vi "new Sub Address.vi"(6 "direction (Tx)":i32(ring) items=["Tx", "Rx"], 7 "messageBufferIDRef (-1)":i32=-1, 8 "error in":errorcluster, 9 "subAddress":i8, 10 "SubAddress Config":T1 {"elapseMinOrMax" items=["A", "B", "AB", "None"]; "timeOrHitCount" items=["Time", "HitCount"]; "dataWipe" items=["Simulate", "Monitor", "Disable"]}, 11 "name":string) -> (0 "error out":errorcluster, 2 "ID out":i32, 3 "subAddress out":refnum<k24>)   [LabVIEW 2020, in "Ballard_1553_Hardware_ni.lvlib"]
uses:
  Ballard_1553_Hardware_ni.lvlib
  C:/Users/Administrator/Desktop/GIT/Ballard-MIL-STD-1553-Custom-Device/Source/System Explorer/SubVIs/Parse XML Ballard/1.2/BTIXML_SerDes.dll
  Ballard-MIL-STD-1553-Custom-Device/Source/System Explorer/SubVIs/Parse XML Ballard/1.2/BTIXML_SerDes.dll
  _typedefs/subAddress_type.ctl
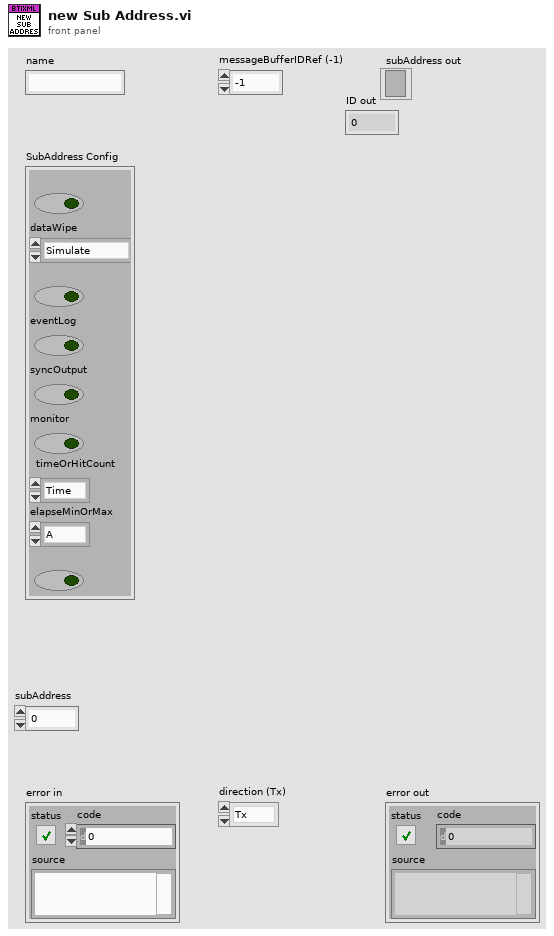
[diagram p1: front panel]
types:
  T1 = typedef "Ballard_1553_Hardware_ni.lvlib/subAddress_type.ctl" = cluster{"enable":bool, "dataWipe":i32, "allowErrorInjection":bool, "eventLog":bool, "syncOutput":bool, "monitor":bool, "timeOrHitCount":i32, "elapseMinOrMax":i32, "wrap":bool}
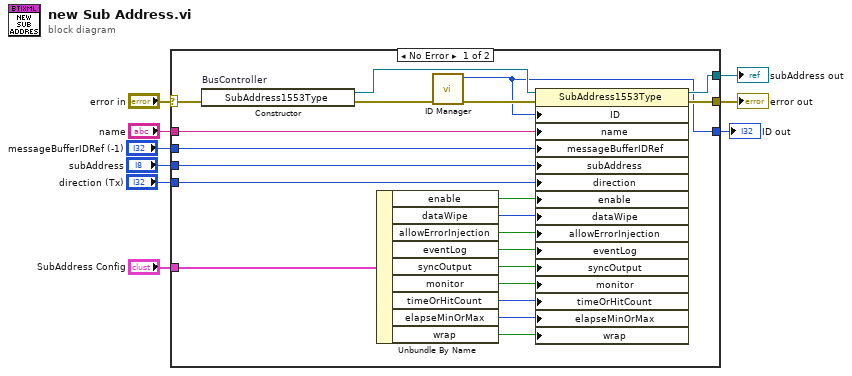
[diagram p0: block diagram]
diagram:
  n1 = case shown="No Error" "error in" {
    selector: "error in" -> [w30 w31]
    tunnel: [w29 w31] -> w8
    tunnel: [w28 _] -> w2
    tunnel: "SubAddress Config" -> [w24 _]
    tunnel: "name" -> [w23 _]
    tunnel: "direction (Tx)" -> [w22 _]
    tunnel: "subAddress" -> [w21 _]
    tunnel: "messageBufferIDRef (-1)" -> [w20 _]
    tunnel: [w10 _] -> w1
    frame No Error {
      n2 = constructor on="BusController" class="SubAddress1553Type"(error in=w30) -> (reference out=w27:refnum<k24>, error out=w26:errorcluster)  [unwired: 2 in, 1 out]
      n3 = Unbundle By Name(w24) -> ("enable"=w19:bool, "dataWipe"=w18:i32, "allowErrorInjection"=w17:bool, "eventLog"=w16:bool, "syncOutput"=w15:bool, "monitor"=w14:bool, "timeOrHitCount"=w13:i32, "elapseMinOrMax"=w12:i32, "wrap"=w11:bool)
      n4 = call "ID Manager.vi"("error in"=w26) -> ("error out"=w25:errorcluster, "ID out"=w10:i32)  [unwired: 9 in]
      n5 = property class="SubAddress1553Type"(reference=w27, error in=w25, "ID"=w10, "name"=w23, "messageBufferIDRef"=w20, "subAddress"=w21, "direction"=w22, "enable"=w19, "dataWipe"=w18, "allowErrorInjection"=w17, "eventLog"=w16, "syncOutput"=w15, "monitor"=w14, "timeOrHitCount"=w13, "elapseMinOrMax"=w12, "wrap"=w11) -> (reference out=w28:refnum<k24>, error out=w29:errorcluster)
    }
    frame Error {
    }
  }
  "error out" <- w8
  "subAddress out" <- w2
  "ID out" <- w1
